vi "Normalization.vi"(1 "Normalize Data":bool, 2 "Array in":dbl[](array[numeric])) -> (0 "Array out":dbl[](array[numeric]))   [LabVIEW 2023]
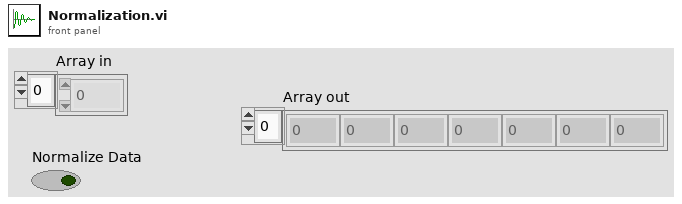
[diagram p1: front panel]
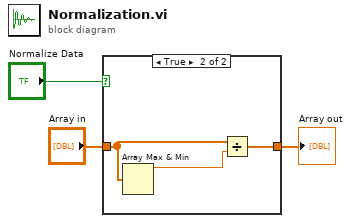
[diagram p0: block diagram]
diagram:
  n1 = case shown="True" "Normalize Data" {
    tunnel: "Array in" -> [w4 w6]
    tunnel: [w4 w5] -> w3
    frame False {
    }
    frame True {
      n2 = Array Max & Min(array=w6) -> (max value=w7:dbl)  [unwired: 3 out]
      n3 = Divide(x=w6, y=w7) -> (x/y=w5:dbl[])
    }
  }
  "Array out" <- w3
